vi "HardwareTimedPulse.vi"(10 "Wait Duration (us)":dbl, 11 "Pulse Duration (us)":dbl) -> ()   [LabVIEW 2009]
uses:
  <vilib>/DAQmx/write.llb/DAQmx Write (Digital Wfm 1Chan NSamp).vi
  <vilib>/DAQmx/configure/timing.llb/DAQmx Timing (Sample Clock).vi
  <vilib>/Waveform/DWDTOps.llb/DWDT Digital Size.vi
  <vilib>/Waveform/DWDTOps.llb/DWDT Append Digital Samples.vi
  <vilib>/Waveform/DWDTOps.llb/Digital Pattern Generator (Single Value).vi
  <vilib>/DAQmx/create/channels.llb/DAQmx Create Channel (DO-Digital Output).vi
panel:
  out "number of samples written per channel":u32
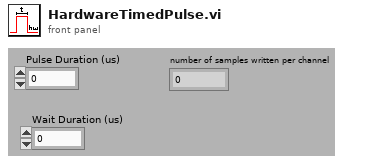
[diagram p1: front panel]
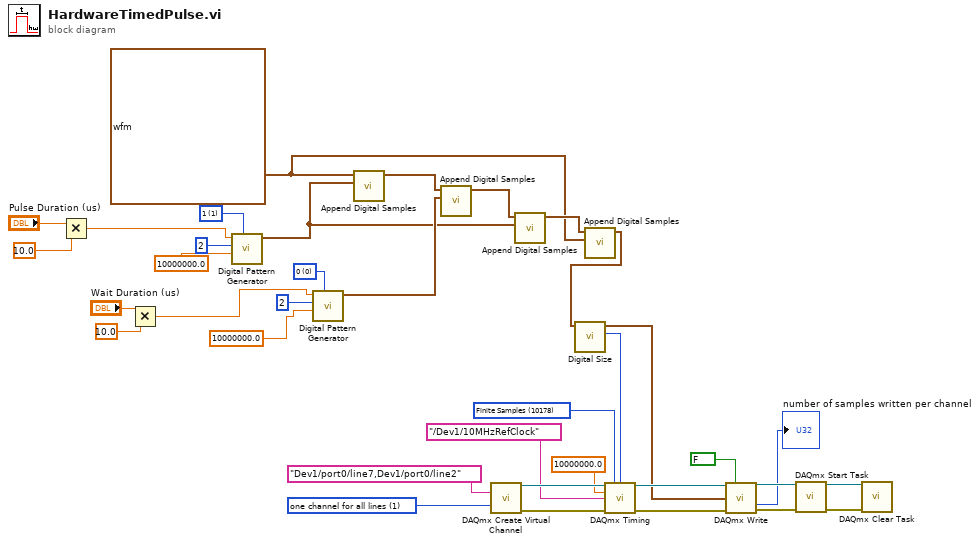
[diagram p0: block diagram]
diagram:
  w12 = u8 0 items=["0", "1", "Z", "L", "H", "X", "T", "V"] ("value")
  w13 = 1 items=["one channel for each line", "one channel for all lines"] ("line grouping")
  w22 = u8 1 items=["0", "1", "Z", "L", "H", "X", "T", "V"] ("value")
  w2 = digitalwaveform {"t0"=timestamp(0 s since 1904-01-01), "dt"=0.0, "Y"={"transitions"=[], "data"=[[0, 0]]}, "error"={"status"=FALSE, "code"=37421928, "source"=""}} ("data")
  w31 = 10178 items=["Finite Samples"=10178, "Continuous Samples"=10123, "Hardware Timed Single Point"=12522] ("sample mode")
  n1 = Multiply(x="Pulse Duration (us)", y=10.0) -> (x*y=w23:dbl)
  n2 = Multiply(x="Wait Duration (us)", y=10.0) -> (x*y=w5:dbl)
  n3 = call-poly <vilib>:"Digital Pattern Generator.vi"("value"=w22, "sample rate"=10000000.0, "number of signals"=u32 2, "number of samples"=w23) -> ("digital waveform"=w9:digitalwaveform)  [unwired: 6 in, 1 out]
  n4 = call-poly <vilib>:"Digital Pattern Generator.vi"("value"=w12, "sample rate"=10000000.0, "number of signals"=u32 2, "number of samples"=w5) -> ("digital waveform"=w11:digitalwaveform)  [unwired: 6 in, 1 out]
  n5 = call-poly <vilib>:"Append Digital Samples.vi"("digital waveform B"=w9, "digital waveform A"=w2) -> ("digital waveform out"=w21:digitalwaveform)  [unwired: 8 in, 1 out]
  n6 = call-poly <vilib>:"Append Digital Samples.vi"("digital waveform B"=w11, "digital waveform A"=w21) -> ("digital waveform out"=w10:digitalwaveform)  [unwired: 8 in, 1 out]
  n7 = call-poly <vilib>:"DAQmx Create Virtual Channel.vi"("lines"=tag "Dev1/port0/line7,Dev1/port0/line2", "line grouping"=w13) -> ("task out"=w35:refnum<k21>, "error out"=w34:errorcluster)  [unwired: 12 in]
  n8 = call-poly <vilib>:"Append Digital Samples.vi"("digital waveform B"=w9, "digital waveform A"=w10) -> ("digital waveform out"=w3:digitalwaveform)  [unwired: 8 in, 1 out]
  n9 = call-poly <vilib>:"Append Digital Samples.vi"("digital waveform B"=w2, "digital waveform A"=w3) -> ("digital waveform out"=w1:digitalwaveform)  [unwired: 8 in, 1 out]
  n10 = call-poly <vilib>:"Digital Size.vi"("digital waveform in"=w1) -> ("number of samples"=w20:i32, "digital waveform out"=w19:digitalwaveform)  [unwired: 7 in, 2 out]
  n11 = call-poly <vilib>:"DAQmx Timing.vi"("task/channels in"=w35, "sample mode"=w31, "samples per channel"=w20, "rate"=10000000.0, "source"=tag "/Dev1/10MHzRefClock", "error in"=w34) -> ("task out"=w29:refnum<k21>, "error out"=w28:errorcluster)  [unwired: 8 in]
  n12 = call-poly <vilib>:"DAQmx Write.vi"("task/channels in"=w29, "auto start"=FALSE, "data"=w19, "error in"=w28) -> ("task out"=w18:refnum<k21>, "number of samples written per channel"=→"number of samples written per channel":u32, "error out"=w17:errorcluster)  [unwired: 9 in]
  n13 = call <vilib>:"DAQmx Start Task.vi"("task/channels in"=w18, "error in"=w17) -> ("task out"=w15:refnum<k21>, "error out"=w14:errorcluster)  [unwired: 12 in]
  n14 = call <vilib>:"DAQmx Clear Task.vi"("task in"=w15, "error in"=w14) -> ()  [unwired: 13 in, 1 out]
